vi "NumericCtlCoercionTest.vi"() -> ()   [LabVIEW 2016]
uses:
  main/apis/Setup/GetVI/GetVIByPath.vi
  main/apis/Stimulus/ValueSignal/ValueSignalByPathString.vi
  main/apis/Assert/AssertControlValue/Equal.vi
  main/Drona.lvlib
  main/apis/Setup/GetVI/GetVI.lvlib
  <vilib>/addons/_JKI Toolkits/Caraya/classes/Test/Test.lvclass
  main/apis/Stimulus/ValueSignal/ValueSignal.lvlib
  main/apis/Assert/AssertControlValue/AssertControlValue.lvlib
panel:
  out "error out":errorcluster
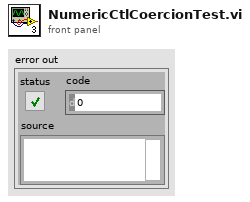
[diagram p1: front panel]
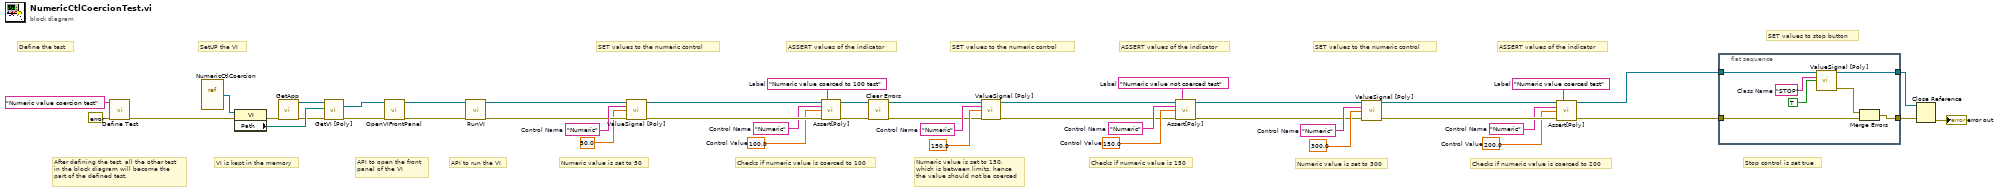
[diagram p0: block diagram]
diagram:
  w5 = "Numeric"  # Control Name
  w7 = "Numeric value coerced test"  # Label
  w8 = 200.0  # Control Value
  w6 = "Numeric"  # Control Name
  w29 = "Numeric"  # Control Name
  w27 = "Numeric value not coerced test"  # Label
  w26 = 150.0  # Control Value
  w28 = "Numeric"  # Control Name
  w32 = "Numeric"  # Control Name
  w35 = "Numeric value coerced to 100 test"  # Label
  w36 = 100.0  # Control Value
  w34 = "Numeric"  # Control Name
  # "Checks if numeric value is coerced to 200"
  # "ASSERT values of the indicator"
  # "Numeric value is set to 300"
  # "SET values to the numeric control"
  # "API to open the front\npanel of the VI"
  # "Stop control is set true"
  # "SET values to stop button"
  # "Checks if numeric value is 150"
  # "ASSERT values of the indicator"
  # "Numeric value is set to 150, \nwhich is between limits, hence\nthe value should not be coerced"
  # "SET values to the numeric control"
  # "Checks if numeric value is coerced to 100"
  # "ASSERT values of the indicator"
  # "Numeric value is set to 50"
  # "API to run the VI"
  # "SET values to the numeric control"
  # "VI is kept in the memory"
  # "SetUP the VI"
  # "After defining the test, all the other test\nin the block diagram will become the \npart of the defined test."
  # "Define the test"
  n1 = call <vilib>:"Define Test.vi"("error in (no error)"=errorcluster {"status"=FALSE, "code"=0, "source"=""}, "Label (VI Title)"="Numeric value coercion test") -> ("error out"=w40:errorcluster)  [unwired: 9 in]
  n2 = vi-ref "NumericCtlCoercion.vi"() -> (w33:refnum<vi>)
  n3 = property on="Property Node" class="VI"(reference=w33, error in=w40) -> (error out=w44:errorcluster, "Path"=w43:path)  [unwired: 1 out]
  n4 = call "GetApp.vi"("error in (no error)"=w44) -> ("Application Ref"=w45:refnum<vi>, "error out"=w42:errorcluster)  [unwired: 13 in]
  n5 = call-poly "GetVI [Poly].vi"("Application Ref in"=w45, "VI Path"=w43, "error in (no error)"=w42) -> ("VI Reference"=w18:refnum<vi>, "error out"=w20:errorcluster)  [unwired: 10 in, 1 out]
  n6 = call "OpenVIFrontPanel.vi"("VI Reference In"=w18, "error in"=w20) -> ("VI Reference Out"=w17:refnum<vi>, "error out"=w19:errorcluster)  [unwired: 12 in]
  n7 = call "RunVI.vi"("VI Reference In"=w17, "error in"=w19) -> ("VI Reference Out"=w31:refnum<vi>, "error out"=w30:errorcluster)  [unwired: 12 in]
  n8 = call-poly "ValueSignal [Poly].vi"("VI Reference In"=w31, "Control Path"=w34, "Value (Signaling)"=50.0, "error in"=w30) -> ("VI Reference Out"=w37:refnum<vi>, "error out"=w38:errorcluster)  [unwired: 10 in]
  n9 = call-poly "Assert[Poly].vi"("VI Reference In"=w37, "Label"=w35, "Control Path"=w32, "Control Value"=w36, "Error In"=w38) -> ("VI Reference Out"=w22:refnum<vi>, "Error Out"=w23:errorcluster)  [unwired: 9 in]
  n10 = call <vilib>:"Clear Errors.vi"("error in (no error)"=w23) -> ("error out"=w14:errorcluster)  [unwired: 5 in, 1 out]
  n11 = call-poly "ValueSignal [Poly].vi"("VI Reference In"=w22, "Control Path"=w28, "Value (Signaling)"=150.0, "error in"=w14) -> ("VI Reference Out"=w25:refnum<vi>, "error out"=w24:errorcluster)  [unwired: 10 in]
  n12 = call-poly "Assert[Poly].vi"("VI Reference In"=w25, "Label"=w27, "Control Path"=w29, "Control Value"=w26, "Error In"=w24) -> ("VI Reference Out"=w1:refnum<vi>, "Error Out"=w4:errorcluster)  [unwired: 9 in]
  n13 = call-poly "ValueSignal [Poly].vi"("VI Reference In"=w1, "Control Path"=w6, "Value (Signaling)"=300.0, "error in"=w4) -> ("VI Reference Out"=w9:refnum<vi>, "error out"=w10:errorcluster)  [unwired: 10 in]
  n14 = call-poly "Assert[Poly].vi"("VI Reference In"=w9, "Label"=w7, "Control Path"=w5, "Control Value"=w8, "Error In"=w10) -> ("VI Reference Out"=w2:refnum<vi>, "Error Out"=w3:errorcluster)  [unwired: 9 in]
  n15 = flat-sequence {
    tunnel: [w49] -> w13
    tunnel: [w50] -> w12
    tunnel: w2 -> [w48]
    tunnel: w3 -> [w46]
    frame #0 {
      w52 = "STOP"  # Class Name
      n16 = call-poly "ValueSignal [Poly].vi"("VI Reference In"=w48, "Control Path"=w52, "Value (Signaling)"=TRUE) -> ("VI Reference Out"=w50:refnum<vi>, "error out"=w47:errorcluster)  [unwired: 11 in]
      n17 = Merge Errors(w47, w46) -> (w49:errorcluster)
    }
  }
  n18 = Close Reference(reference=w12, error in (no error)=w13) -> (error out=→"error out":errorcluster)
